vi "PPDA Partial Pressure of Dry Air in Humid Air(Pa).vi"(1 "Total Pressure of Humid Air":dbl[unit], 2 "Tceg":dbl[unit], 3 "RH":dbl) -> (0 "PPDA":dbl[unit])   [LabVIEW 2018]
panel:
  out "Humidity of Input Air":dbl(knob) scale=0.0..100.0
  out "PPDA \nPartial Pressure of Dry Air in Humid Air(Pa)\nPPDA=Ptotal-PPWV":dbl[unit](knob)
  out "Temprature Of Input Air\nCentigrade Degree":dbl[unit](slide) scale=0.0..100.0
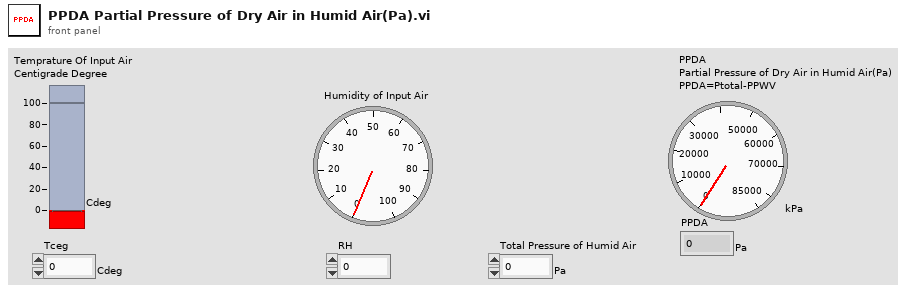
[diagram p1: front panel]
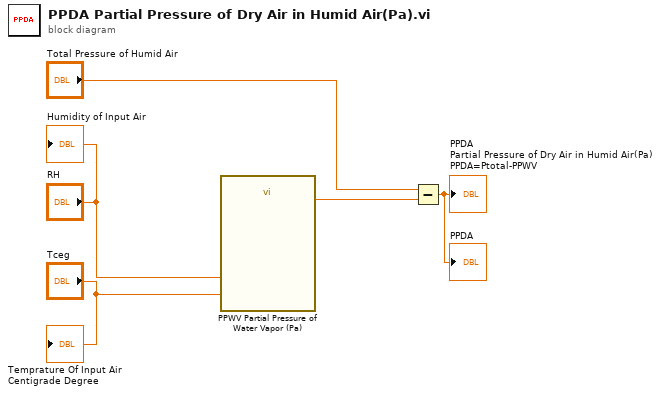
[diagram p0: block diagram]
diagram:
  n1 = call "PPWV Partial Pressure of Water Vapor (Pa).vi"("Tceg"="Tceg", "RH"="RH") -> ("PPWV"=w4:dbl[unit])
  n2 = Subtract(x="Total Pressure of Humid Air", y=w4) -> (x-y=→"PPDA \nPartial Pressure of Dry Air in Humid Air(Pa)\nPPDA=Ptotal-PPWV" →"PPDA":dbl[unit])
  "Temprature Of Input Air\nCentigrade Degree" <- "Tceg"
  "Humidity of Input Air" <- "RH"
